vi "Set SSR Status - All.vi"(0 "reference in":refnum<class "SSR.lvclass">, 4 "All SSR On/Off":bool, 5 "error in (no error)":errorcluster) -> (14 "reference out":refnum<class "SSR.lvclass">, 19 "error out":errorcluster)   [LabVIEW 2017, in "SSR.lvclass"]
uses:
  SSR.lvclass
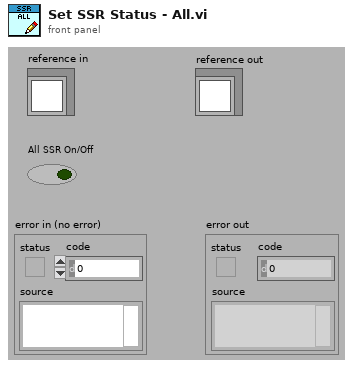
[diagram p1: front panel]
types:
  T1 = typedef "SSR.lvclass/ObjectAttributes.ctl" = cluster{"SSR Task":refnum<k21>, "SSR On/Off Status":bool, "Number of SSR Modules":u32, "Number of Total SSR Channels":u32, "SSR Module Names (NI-Max Name)":string[], "Number of Channels Per SSR Module":i32[], "SSR Status":bool[], "SSR Status to Set":bool[], "SSR VI Reference":refnum<vi>}
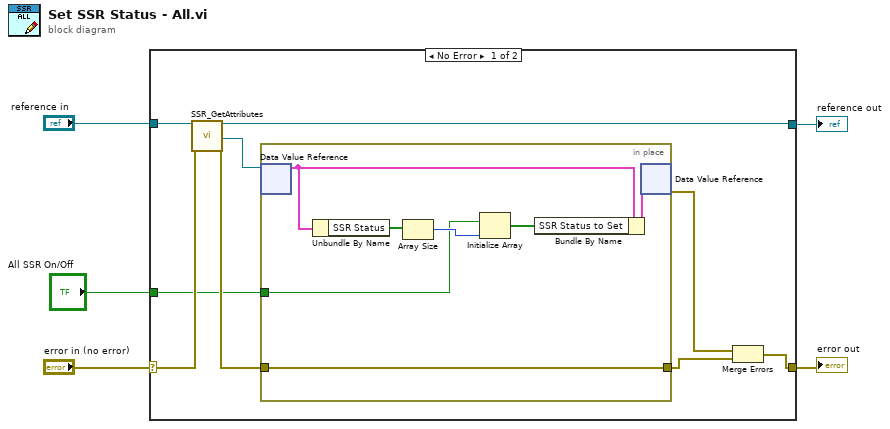
[diagram p0: block diagram]
diagram:
  n1 = case shown="No Error" "error in (no error)" {
    selector: "error in (no error)" -> [w13 w23]
    tunnel: [w10 w23] -> w4
    tunnel: [w11 w22] -> w2
    tunnel: "reference in" -> [w14 w22]
    tunnel: "All SSR On/Off" -> [w6 _]
    frame No Error {
      n2 = call "SSR_GetAttributes.vi"("reference in"=w14, "error in (no error)"=w13) -> ("reference out"=w11:refnum<class "SSR.lvclass">, "DataRef"=w9:refnum<data-value>, "error out"=w8:errorcluster)  [unwired: 14 in, 1 out]
      n3 = in-place {
        in-place-border: w8 -> [w19]
        in-place-border: [w19] -> w7
        in-place-border: w6 -> [w16]
        n4 = in-place-dvr #1(w9) -> (w20:T1)  [unwired: 1 out]
        n5 = Unbundle By Name(w20) -> ("SSR Status"=w18:bool[])
        n6 = Array Size(array=w18) -> (size(s)=w17:i32)
        n7 = Initialize Array(w16, w17) -> (w15:bool[])
        n8 = Bundle By Name(cluster=w20, "SSR Status to Set"=w15) -> (w21:T1)
        n9 = in-place-dvr #1(w21) -> (w12:errorcluster)  [unwired: 1 out]
      }
      n10 = Merge Errors(w12, w7) -> (w10:errorcluster)
    }
    frame Error {
    }
  }
  "error out" <- w4
  "reference out" <- w2
